vi "get datasets from modules.vi"(8 "error in":errorcluster, 11 "Modules Configurations":refnum<class "TBM module configuration.lvclass">[](array[class])) -> (0 "error out":errorcluster, 3 "module datasets":T1[](array[typedef]))   [LabVIEW 2013, in "PL Framework Configuration Tool.lvlib" / "Engine Mappings.lvclass"]
uses:
  Engine Mappings.lvclass
  <vilib>/NI/Tag Bus Module Framework/module configuration/TBM module configuration.lvclass
  module information.ctl
  <vilib>/NI/Tag Bus Module Framework/channel/TBM channel.lvclass
  <vilib>/NI/Configuration Framework/serializable configuration/NISE_CEF_serializable configuration.lvclass/NISE_CEF_serializable configuration.ctl
  <vilib>/NI/Configuration Framework/error generator/NISE_error generator.vi
  <vilib>/NI/Configuration Framework/serializable configuration/NISE_CEF_serializable configuration.lvclass
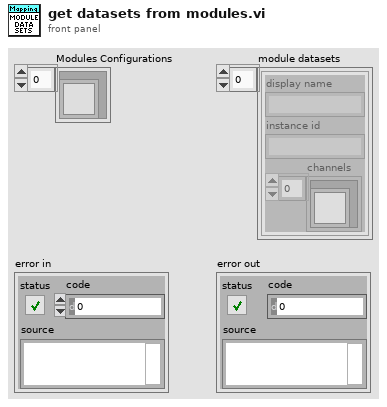
[diagram p1: front panel]
types:
  T1 = typedef "PL Framework Configuration Tool.lvlib/Engine Mappings.lvclass/module information.ctl" = cluster{"display name":string, "instance id":string, "channels":refnum<class "TBM channel.lvclass">[]}
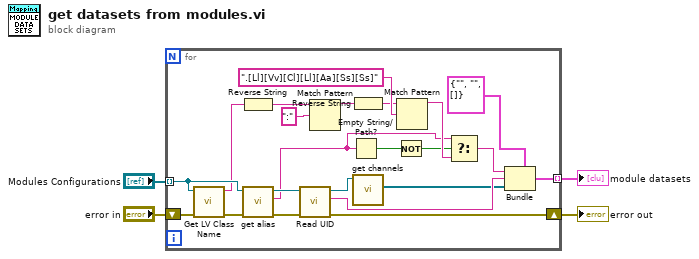
[diagram p0: block diagram]
diagram:
  n1 = for {
    shift-right: [w9] -> w2
    shift-left: "error in" -> [w24]
    tunnel: "Modules Configurations" -> [w22] mode=indexing
    tunnel: [w8] -> w1 mode=indexing
    n2 = call <vilib>:"Get LV Class Name.vi"("error in (no error)"=w24, "object"=w22) -> ("error out"=w23:errorcluster, "class name"=w18:string)  [unwired: 8 in]
    n3 = Reverse String(1:w18) -> (0:w17:string)
    n4 = call <vilib>:"get alias.vi"("error in"=w23, "configuration in"=w22) -> ("error out"=w25:errorcluster, "alias"=w5:string, "configuration out"=w26:refnum<class "TBM module configuration.lvclass">)  [unwired: 7 in]
    n5 = call <vilib>:"Read UID.vi"("error in"=w25, "configuration in"=w26) -> ("error out"=w9:errorcluster, "instance id"=w13:string, "configuration out"=w12:refnum<class "TBM module configuration.lvclass">)  [unwired: 7 in]
    n6 = Match Pattern(string=w17, regular expression=":") -> (before substring=w16:string)  [unwired: 1 in, 3 out]
    n7 = Empty String/Path?(string/path=w5) -> (empty?=w7:bool)
    n8 = Reverse String(1:w16) -> (0:w15:string)
    n9 = call-dynamic "get channels.vi"("module configuration in"=w12) -> ("channels"=w11:refnum<class "TBM channel.lvclass">[])  [unwired: 9 in, 1 out]
    n10 = Not(x=w7) -> (.not. x?=w6:bool)
    n11 = Match Pattern(string=w15, regular expression=".[Ll][Vv][Cl][Ll][Aa][Ss][Ss]") -> (before substring=w20:string)  [unwired: 1 in, 3 out]
    n12 = Select(t=w5, s=w6, f=w20) -> (s? t:f=w14:string)
    n13 = Bundle(cluster=T1 {"display name"="", "instance id"="", "channels"=[]} ("module info"), "display name"=w14, "instance id"=w13, "channels"=w11) -> (w8:T1)
  }
  "error out" <- w2
  "module datasets" <- w1
